vi "diceRoll.vi"(3 "Roll Button":bool) -> (0 "player2":dbl, 1 "player1":dbl)   [LabVIEW 2014]
doc: "Randomly rolls a dice for each player, when player1 or player2 push the roll buttons on top VI."
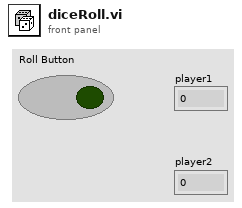
[diagram p1: front panel]
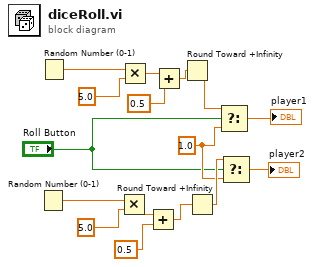
[diagram p0: block diagram]
diagram:
  w8 = 1.0
  n1 = Random Number (0-1)() -> (number: 0 to 1=w14:dbl)
  n2 = Random Number (0-1)() -> (number: 0 to 1=w16:dbl)
  n3 = Multiply(x=w14, y=5.0) -> (x*y=w4:dbl)
  n4 = Multiply(x=w16, y=5.0) -> (x*y=w6:dbl)
  n5 = Add(x=w4, y=0.5) -> (x+y=w2:dbl)
  n6 = Add(x=w6, y=0.5) -> (x+y=w1:dbl)
  n7 = Round Toward +Infinity(x=w1) -> (ceil(x): smallest int >= x=w12:dbl)
  n8 = Round Toward +Infinity(x=w2) -> (ceil(x): smallest int >= x=w10:dbl)
  n9 = Select(t=w12, s="Roll Button", f=w8) -> (s? t:f=→"player1":dbl)
  n10 = Select(t=w10, s="Roll Button", f=w8) -> (s? t:f=→"player2":dbl)
